vi "wfg.vi"(0 "reference in":refnum<class "Timer.lvclass">, 5 "error in (no error)":errorcluster) -> (14 "reference out":refnum<class "Timer.lvclass">, 19 "error out":errorcluster)   [LabVIEW 2017, in "Timer.lvclass"]
uses:
  Timer.lvclass
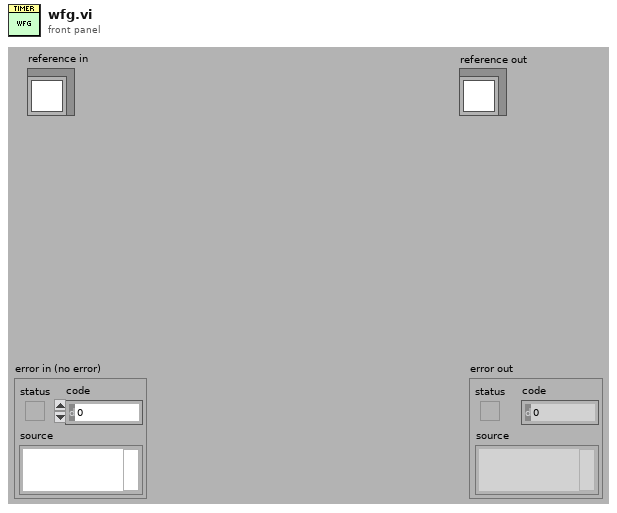
[diagram p1: front panel]
types:
  T1 = typedef "Timer.lvclass/ObjectAttributes.ctl" = cluster{"Timer is Timing":bool, "Timer Time (ms)":u32, "Timer VI Reference":refnum<vi>}
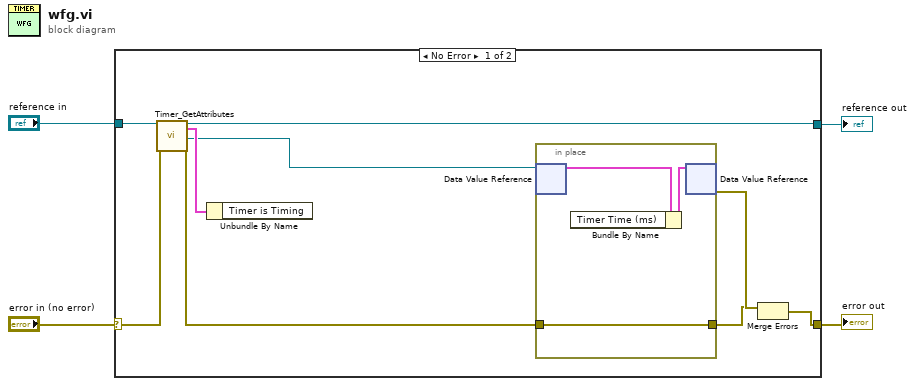
[diagram p0: block diagram]
diagram:
  n1 = case shown="No Error" "error in (no error)" {
    selector: "error in (no error)" -> [w12 w18]
    tunnel: [w8 w18] -> w3
    tunnel: [w9 w17] -> w1
    tunnel: "reference in" -> [w13 w17]
    frame No Error {
      n2 = call "Timer_GetAttributes.vi"("reference in"=w13, "error in (no error)"=w12) -> ("reference out"=w9:refnum<class "Timer.lvclass">, "Data"=w11:T1, "DataRef"=w7:refnum<data-value>, "error out"=w6:errorcluster)  [unwired: 14 in]
      n3 = Unbundle By Name(w11) -> ()  [unwired: 1 out]
      n4 = in-place {
        in-place-border: w6 -> [w14]
        in-place-border: [w14] -> w5
        n5 = in-place-dvr #1(w7) -> (w15:T1)  [unwired: 1 out]
        n6 = Bundle By Name(cluster=w15) -> (w16:T1)  [unwired: 1 in]
        n7 = in-place-dvr #1(w16) -> (w10:errorcluster)  [unwired: 1 out]
      }
      n8 = Merge Errors(w10, w5) -> (w8:errorcluster)
    }
    frame Error {
    }
  }
  "error out" <- w3
  "reference out" <- w1
